vi "test_Import Configuration_Group.vi"(8 "error in (no error)":errorcluster, 11 "TestCase in":refnum<class "FPGA Addon Scripting API Unit Tests.lvclass">=refnum) -> (0 "error out":errorcluster, 3 "TestCase out":refnum<class "FPGA Addon Scripting API Unit Tests.lvclass">)   [LabVIEW 2026, in "FPGA Addon Scripting API Unit Tests.lvclass"]
uses:
  FPGA Addon Scripting API Unit Tests.lvclass
  FPGA Addon Test Class/FPGA Addon Test Class.lvclass
  APIs/Scripting API/Scripting API.lvlib
  APIs/Scripting API/TypeDefs/Output Scalar Data.ctl
  Addon/Addon Shared/Types/FPGA Addon Data Type.ctl
  Addon/Addon Shared/FPGA Addon Shared.lvlib
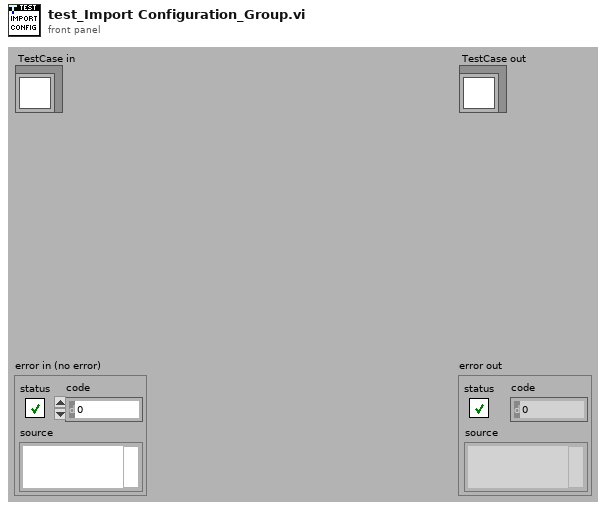
[diagram p1: front panel]
types:
  T1 = typedef "Scripting API.lvlib/Output Scalar Data.ctl" = cluster{"Bitfile Name":string, "SysDef Channel Name":string, "Imported":bool, "Data Type":T2}
  T2 = typedef "FPGA Addon Shared.lvlib/FPGA Addon Data Type.ctl" = enum8{"<Null>", "I8", "I16", "I32", "I64", "U8", "U16", "U32", "U64", "SGL", "Boolean", "Analog PWM In Settings", "Analog PWM In", "Digital PWM In Settings", "Digital PWM In", "Digital PWM Out", "Sine Out", "FXP", "FXP+/-24.5", "FXP+/-16.5", "FXP+/-32.8", "FXP+/-64.32", "FXP+/-16.7", "FXP+/-20.5", "FXP+/-27.5", "FXP+/-32.16", "FXP+16.3", "FXP+18.3", "Digital Static In", "Digital Static Out", "Digital Static In Settings", "Digital WSS Out", "Quad Encoder Settings", "Quad Encoder In", "Group"}
  T3 = typedef "Custom Device API.lvlib/Custom Device Item Ref.ctl" = u64
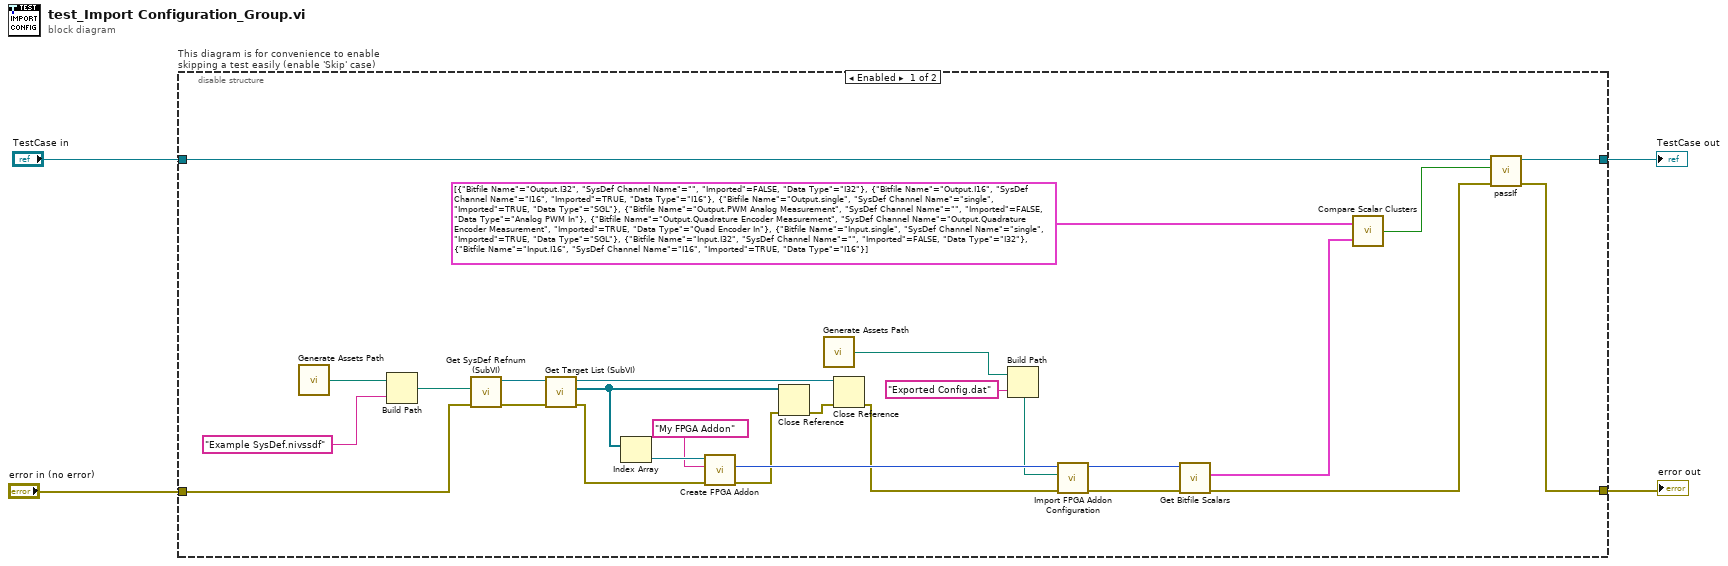
[diagram p0: block diagram]
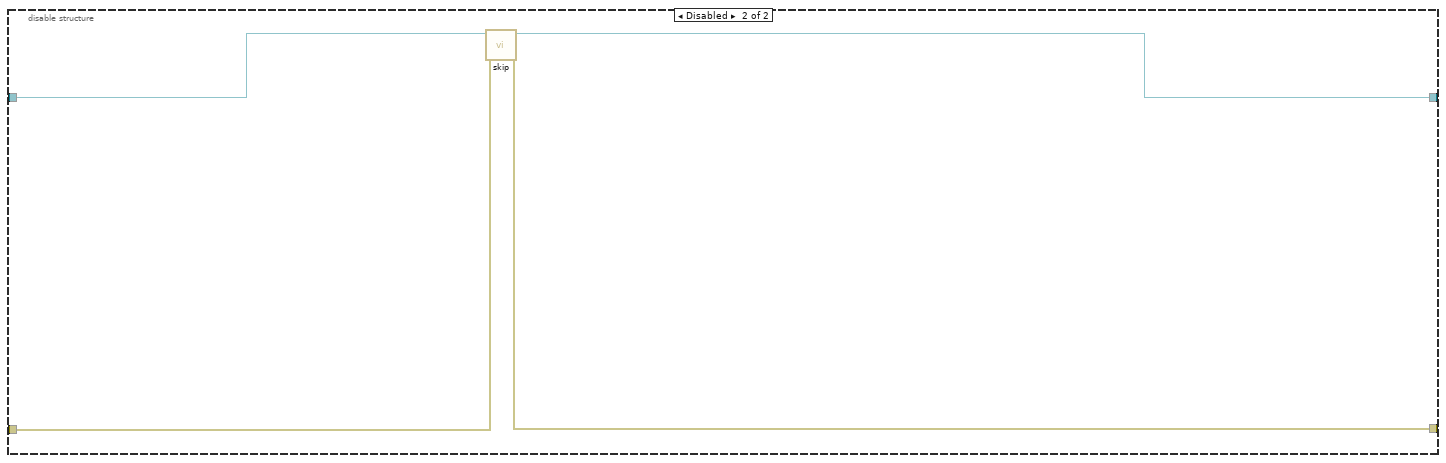
[diagram p2: hidden frame]
diagram:
  n1 = disable-structure "This diagram is for convenience to enable skipping a test easily (enable 'Skip' case)" shown="Enabled" {
    disable-tunnel: "TestCase in" -> [w11 w35]
    disable-tunnel: [w8 w33] -> w1
    disable-tunnel: [w9 w34] -> w3
    disable-tunnel: "error in (no error)" -> [w27 w32]
    frame Enabled {
      n2 = call "Generate Assets Path.vi"() -> ("Assets path"=w31:path)
      n3 = Build Path(base path=w31, name or relative path="Example SysDef.nivssdf") -> (appended path=w29:path)
      n4 = call "Get SysDef Refnum (SubVI).vi"("error in (no error)"=w27, "System Definition path"=w29) -> ("error out"=w26:errorcluster, "NationalInstruments.VeriStand.SystemDefinitionAPI.SystemDefinition"=w28:refnum<k39>)  [unwired: 8 in]
      n5 = call "Get Target List (SubVI).vi"("error in (no error)"=w26, "NationalInstruments.VeriStand.SystemDefinitionAPI.SystemDefinition"=w28) -> ("error out"=w25:errorcluster, "Target List Refnums"=w15:refnum<k39>[], "NationalInstruments.VeriStand.SystemDefinitionAPI.SystemDefinition"=w16:refnum<k39>)  [unwired: 7 in]
      n6 = Index Array(array=w15) -> (element=w24:refnum<k39>)  [unwired: 1 in]
      n7 = call "Create FPGA Addon.vi"("error in"=w25, "FPGA addon name"="My FPGA Addon", "NationalInstruments.VeriStand.SystemDefinitionAPI.Target"=w24) -> ("error out"=w14:errorcluster, "FPGA addon refnum"=w22:T3)  [unwired: 6 in, 1 out]
      n8 = Close Reference(reference=w15, error in (no error)=w14) -> (error out=w13:errorcluster)
      n9 = call "Generate Assets Path.vi"() -> ("Assets path"=w21:path)
      n10 = Close Reference(reference=w16, error in (no error)=w13) -> (error out=w12:errorcluster)
      n11 = Build Path(base path=w21, name or relative path="Exported Config.dat") -> (appended path=w19:path)
      n12 = call "Import FPGA Addon Configuration.vi"("error in"=w12, "configuration file path"=w19, "FPGA addon refnum in"=w22) -> ("error out"=w18:errorcluster, "FPGA addon refnum out"=w17:T3)  [unwired: 7 in]
      n13 = call "Get Bitfile Scalars.vi"("error in"=w18, "FPGA addon refnum in"=w17) -> ("error out"=w10:errorcluster, "bitfile scalars out"=w7:T1[])  [unwired: 7 in, 1 out]
      n14 = call "Compare Scalar Clusters.vi"("Target bitfile scalars in"=w7, "Reference bitfile scalars in"=T1[] [{"Bitfile Name"="Output.I32", "SysDef Channel Name"="", "Imported"=FALSE, "Data Type"=enum."I32"}, {"Bitfile Name"="Output.I16", "SysDef Channel Name"="I16", "Imported"=TRUE, "Data Type"=enum."I16"}, {"Bitfile Name"="Output.single", "SysDef Channel Name"="single", "Imported"=TRUE, "Data Type"=enum."SGL"}, {"Bitfile Name"="Output.PWM Analog Measurement", "SysDef Channel Name"="", "Imported"=FALSE, "Data Type"=enum."Analog PWM In"}, {"Bitfile Name"="Output.Quadrature Encoder Measurement", "SysDef Channel Name"="Output.Quadrature Encoder Measurement", "Imported"=TRUE, "Data Type"=enum."Quad Encoder In"}, {"Bitfile Name"="Input.single", "SysDef Channel Name"="single", "Imported"=TRUE, "Data Type"=enum."SGL"}, {"Bitfile Name"="Input.I32", "SysDef Channel Name"="", "Imported"=FALSE, "Data Type"=enum."I32"}, {"Bitfile Name"="Input.I16", "SysDef Channel Name"="I16", "Imported"=TRUE, "Data Type"=enum."I16"}] ("bitfile scalars out")) -> ("Equal ?"=w5:bool)
      n15 = call-dynamic "passIf.vi"("error in (no error)"=w10, "pass"=w5, "TestCase in"=w11) -> ("error out"=w9:errorcluster, "TestCase out"=w8:refnum<class "FPGA Addon Scripting API Unit Tests.lvclass">)  [unwired: 7 in]
    }
    frame Disabled {
      # "skip test result while test is under development"
      n16 = call <vilib>:"skip.vi"("error in (no error)"=w32, "TestCase in"=w35) -> ("error out"=w34:errorcluster, "TestCase out"=w33:refnum<class "FPGA Addon Scripting API Unit Tests.lvclass">)  [unwired: 8 in]
    }
  }
  "error out" <- w3
  "TestCase out" <- w1
